vi "Create new save file.vi"(2 "Insert":string, 3 "Ext":string=".dat", 4 "Index In":dbl=1.0) -> (0 "Path Out":path, 1 "Index Out":dbl)   [LabVIEW 2016]
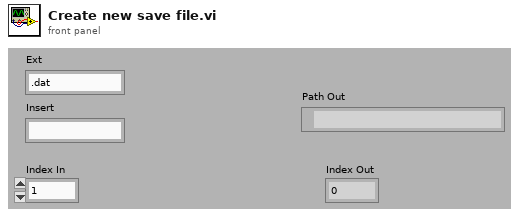
[diagram p1: front panel]
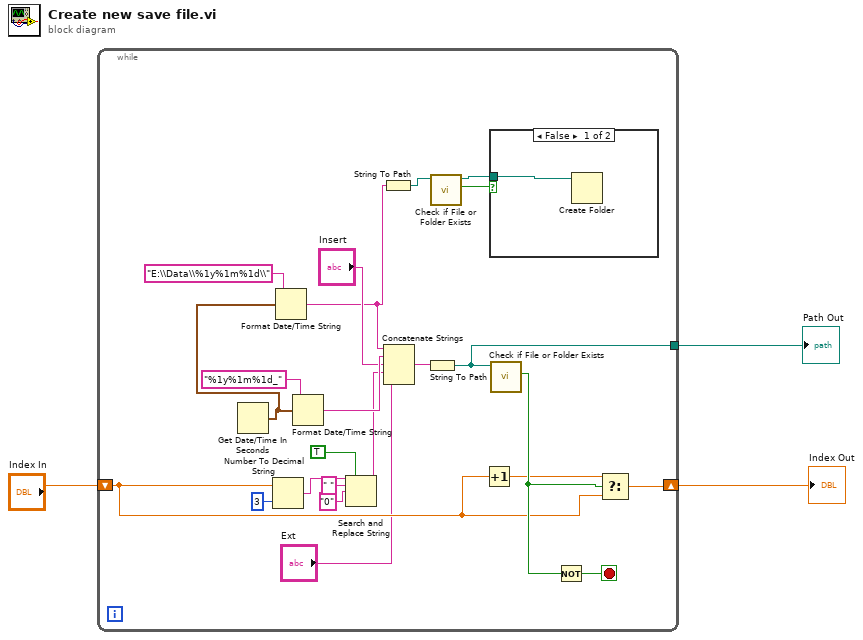
[diagram p0: block diagram]
diagram:
  n1 = while {
    tunnel: [w20] -> w2
    shift-right: [w18] -> w1
    shift-left: "Index In" -> [w16]
    stop <- w19 stop-if-true
    n2 = Get Date/Time In Seconds() -> (seconds since 1Jan1904=w11:timestamp)
    n3 = Number To Decimal String(number=w16, width (-)=i16 3) -> (decimal integer string=w22:string)
    n4 = Format Date/Time String(time format string (%c)="E:\\Data\\%1y%1m%1d\\", seconds (now)=w11) -> (date/time string=w7:string)  [unwired: 1 out]
    n5 = Format Date/Time String(time format string (%c)="%1y%1m%1d_", seconds (now)=w11) -> (date/time string=w25:string)  [unwired: 1 out]
    n6 = Search and Replace String(replace all?=TRUE ("replace all? (F)"), input string=w22, search string=" ", replace string="0" ("replace string (\"\")")) -> (result string=w10:string)  [unwired: 1 in, 6 out]
    n7 = String To Path(string=w7) -> (path=w6:path)
    n8 = Concatenate Strings(w7, w25, "Insert", w10, "Ext") -> (w26:string)
    n9 = String To Path(string=w26) -> (path=w20:path)
    n10 = call <vilib>:"Check if File or Folder Exists.vi"("path"=w6) -> ("file or folder exists?"=w5:bool, "dup path"=w4:path)  [unwired: 1 in, 8 out]
    n11 = Increment(x=w16) -> (x+1=w15:dbl)
    n12 = case shown="False" w5 {
      tunnel: w4 -> [w27 _]
      frame False {
        n13 = Create Folder(path (use dialog)=w27) -> ()  [unwired: 1 in, 4 out]
      }
      frame True {
      }
    }
    n14 = call <vilib>:"Check if File or Folder Exists.vi"("path"=w20) -> ("file or folder exists?"=w17:bool)  [unwired: 1 in, 9 out]
    n15 = Not(x=w17) -> (.not. x?=w19:bool)
    n16 = Select(t=w15, s=w17, f=w16) -> (s? t:f=w18:dbl)
  }
  "Index Out" <- w1
  "Path Out" <- w2
